vi "UpdatePath.vi"(7 "File Name Prefix (Optional)":string, 8 "error in (no error)":errorcluster, 9 "Project Root":path, 10 "Project Name":string, 11 "MetaDataObj in":refnum<class "MetaDataObj.lvclass">) -> (0 "error out":errorcluster, 3 "MetaDataObj out":refnum<class "MetaDataObj.lvclass">)   [LabVIEW 2021, in "myRIOMetaDataObj.lvclass"]
uses:
  myRIOMetaDataObj.lvclass
  <resource>/dialog/NewProjectWizard/MetaDataObj/MetaDataObj.lvclass
  <resource>/dialog/NewProjectWizard/MetaDataObj/MetaDataObj.lvclass/MetaDataObj.ctl
  <resource>/dialog/NewProjectWizard/MetaDataObj/Accessors/Write File Prefix.vi
  <resource>/dialog/NewProjectWizard/MetaDataObj/Accessors/Write Project Name.vi
  <resource>/dialog/NewProjectWizard/MetaDataObj/Accessors/Write Project Root.vi
  <resource>/dialog/NewProjectWizard/MetaDataObj/Accessors/Read Hide Prefix.vi
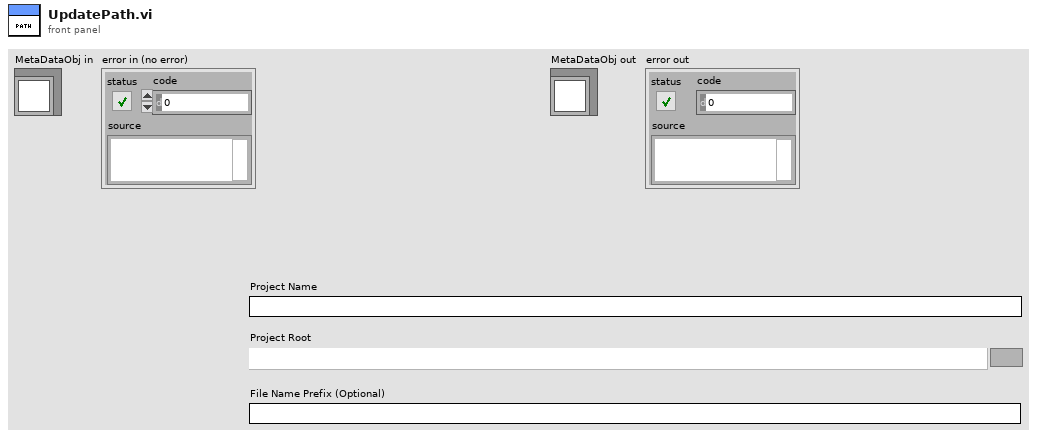
[diagram p1: front panel]
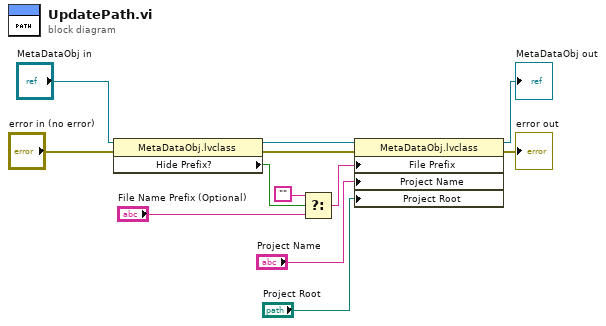
[diagram p0: block diagram]
diagram:
  n1 = property class="MetaDataObj.lvclass"(reference="MetaDataObj in", error in="error in (no error)") -> (reference out=w10:refnum<class "MetaDataObj.lvclass">, error out=w5:errorcluster, "Hide Prefix?"=w8:bool)
  n2 = Select(t="", s=w8, f="File Name Prefix (Optional)") -> (s? t:f=w7:string)
  n3 = property class="MetaDataObj.lvclass"(reference=w10, error in=w5, "File Prefix"=w7, "Project Name"="Project Name", "Project Root"="Project Root") -> (reference out=→"MetaDataObj out":refnum<class "MetaDataObj.lvclass">, error out=→"error out":errorcluster)
